vi "LAC Cmd103_Batch Setting_ver1.vi"(6 "R/W (F:Read)":bool, 7 "timeout(ms)":u32, 8 "error in":errorcluster, 9 "setting_items":T1, 11 "VISA name in":refnum<visa-resource-name>) -> (0 "error out":errorcluster, 1 "read buffer":string, 3 "VISA name out":refnum<visa-resource-name>)   [LabVIEW 8.6]
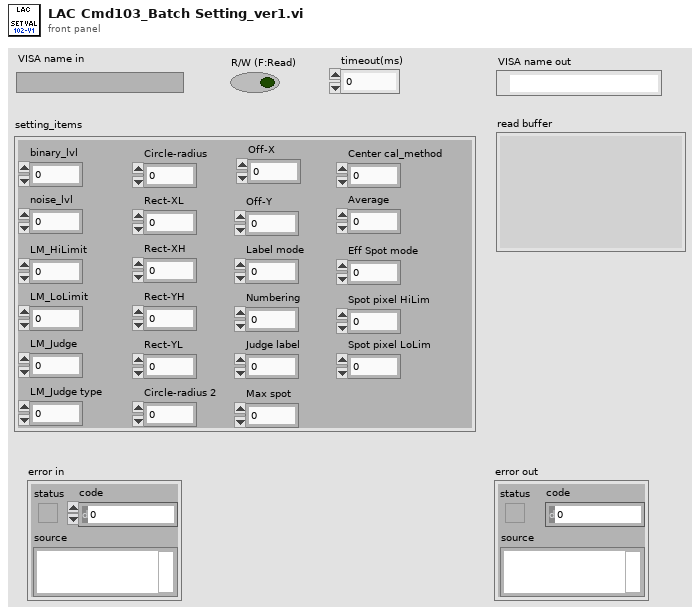
[diagram p1: front panel]
types:
  T1 = cluster{"binary_lvl":u16, "noise_lvl":u16, "LM_HiLimit":u16, "LM_LoLimit":u16, "LM_Judge":u8, "LM_Judge type":u8, "Circle-radius":dbl, "Rect-XL":dbl, "Rect-XH":dbl, "Rect-YH":dbl, "Rect-YL":dbl, "Circle-radius 2":dbl, "Off-X":dbl, "Off-Y":dbl, "Label mode":u8, "Numbering":u8, "Judge label":u8, "Max spot":u8, "Center cal_method":u8, "Average":u8, "Eff Spot mode":u8, "Spot pixel HiLim":u16, "Spot pixel LoLim":u16}
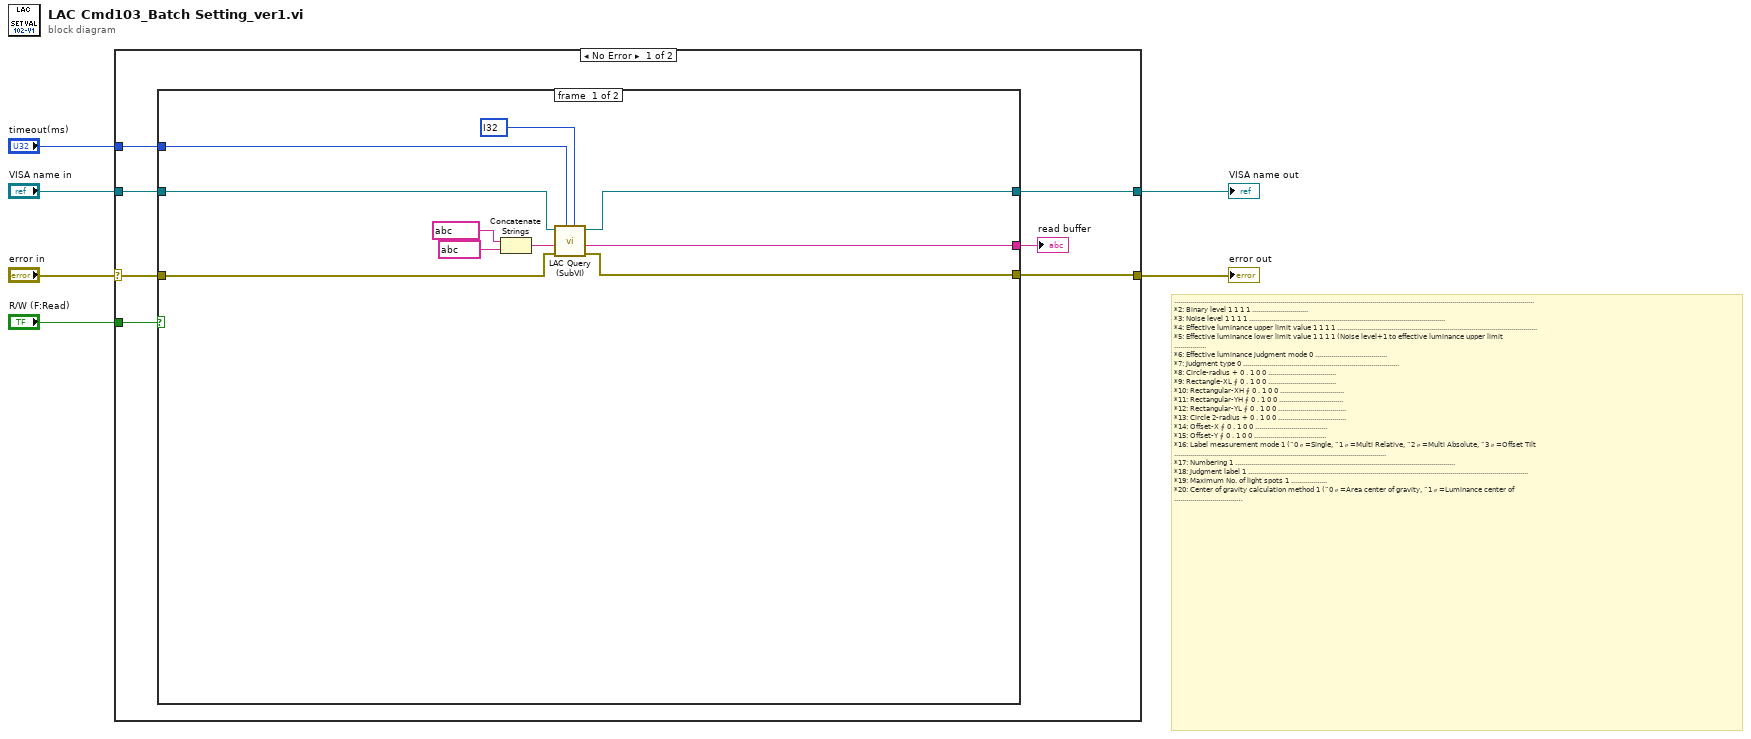
[diagram p0: block diagram]
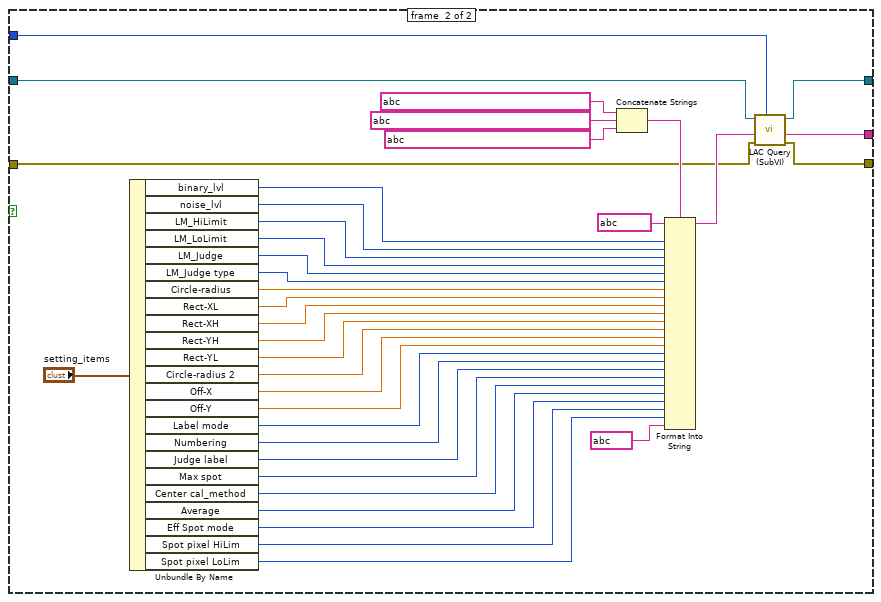
[diagram p2: hidden frame]
diagram:
  # "....................................................................................................................................................................................\n*2: Binary level 1 1 1 1 ............................\n*3: Noise level 1 1 1 1 ..................................................................................................\n*4: Effective luminance upper limit value 1 1 1 1 ....................................................................................................\n*5: Effective luminance lower limit value 1 1 1 1 (Noise level+1 to effective luminance upper limit\n................\n*6: Effective luminance judgment mode 0 ....................................\n*7: Judgment type 0 ..............................................................................\n*8: Circle-radius + 0 . 1 0 0 ..................................\n*9: Rectangle-XL ∮ 0 . 1 0 0 ..................................\n*10: Rectangular-XH ∮ 0 . 1 0 0 ................................\n*11: Rectangular-YH ∮ 0 . 1 0 0 ................................\n*12: Rectangular-YL ∮ 0 . 1 0 0 ..................................\n*13: Circle 2-radius + 0 . 1 0 0 ..................................\n*14: Offset-X ∮ 0 . 1 0 0 ....................................\n*15: Offset-Y ∮ 0 . 1 0 0 ....................................\n*16: Label measurement mode 1 (¨0〃=Single, ¨1〃=Multi Relative, ¨2〃=Multi Absolute, ¨3〃=Offset TIlt\n..........................................................................................................\n*17: Numbering 1 ..............................................................................................................\n*18: Judgment label 1 ............................................................................................................................................\n*19: Maximum No. of light spots 1 ..................\n*20: Center of gravity calculation method 1 (¨0〃=Area center of gravity, ¨1〃=Luminance center of\n........................................................\n*21: Average 1 ..............................................................................................................................\n*22: Effective light spot size mode 1 ....................................\n*23: Effective light spot pixel upper limit value 1 1 1 1 1 1 (Effective light spot pixel lower limit\n..................................\n*24: Effective light spot pixel lower limit value 1 1 1 1 1 1 (1 to Effective light spot pixel upper limit\n................"
  n1 = case shown="No Error" "error in" {
    selector: "error in" -> [w9 w62]
    tunnel: [w12 w61] -> w6
    tunnel: [w11 w62] -> w5
    tunnel: "timeout(ms)" -> [w7 _]
    tunnel: "R/W (F:Read)" -> [w13 _]
    tunnel: "VISA name in" -> [w8 w61]
    frame #0 {
      n2 = case shown="True" w13 {
        tunnel: [w16 w30] -> w11
        tunnel: [w15 w29] -> w12
        tunnel: [w14 w27] -> w10
        tunnel: w9 -> [w19 w26]
        tunnel: w8 -> [w18 w25]
        tunnel: w7 -> [w17 w24]
        frame #0 {
          n3 = Concatenate Strings(string ? ("string"), string ? ("write buffer")) -> (w23:string)
          n4 = call "LAC Query (SubVI).vi"("interval(ms)"=i32 ?, "timeout(ms)"=w17, "error in"=w19, "Command"=w23, "VISA name in"=w18) -> ("error out"=w16:errorcluster, "read buffer"=w14:string, "VISA name out"=w15:refnum<visa-resource-name>)  [unwired: 4 in]
        }
        frame #1 {
          n5 = Unbundle By Name("setting_items") -> ("binary_lvl"=w54:u16, "noise_lvl"=w53:u16, "LM_HiLimit"=w52:u16, "LM_LoLimit"=w51:u16, "LM_Judge"=w50:u8, "LM_Judge type"=w49:u8, "Circle-radius"=w48:dbl, "Rect-XL"=w47:dbl, "Rect-XH"=w46:dbl, "Rect-YH"=w45:dbl, "Rect-YL"=w44:dbl, "Circle-radius 2"=w43:dbl, "Off-X"=w42:dbl, "Off-Y"=w41:dbl, "Label mode"=w40:u8, "Numbering"=w39:u8, "Judge label"=w38:u8, "Max spot"=w37:u8, "Center cal_method"=w36:u8, "Average"=w35:u8, "Eff Spot mode"=w34:u8, "Spot pixel HiLim"=w33:u16, "Spot pixel LoLim"=w32:u16)
          n6 = Concatenate Strings(string ? ("format string"), string ? ("string"), string ? ("format string")) -> (w60:string)
          n7 = Format Into String(format string=w60, initial string=string ? ("string"), w54, w53, w52, w51, w50, w49, w48, w47, w46, w45, w44, w43, w42, w41, w40, w39, w38, w37, w36, w35, w34, w33, w32, string ? ("write buffer")) -> (resulting string=w28:string)  [unwired: 1 in, 1 out]
          n8 = call "LAC Query (SubVI).vi"("timeout(ms)"=w24, "error in"=w26, "Command"=w28, "VISA name in"=w25) -> ("error out"=w30:errorcluster, "read buffer"=w27:string, "VISA name out"=w29:refnum<visa-resource-name>)  [unwired: 5 in]
        }
      }
      "read buffer" <- w10
    }
    frame #1 {
    }
  }
  "VISA name out" <- w6
  "error out" <- w5
